vi "sinusiki 22.vi"(6 "k":dbl, 9 "N":i32, 10 "Faza":dbl, 11 "Amplituda":dbl) -> (3 "Array":dbl[](array[numeric]))   [LabVIEW 2020]
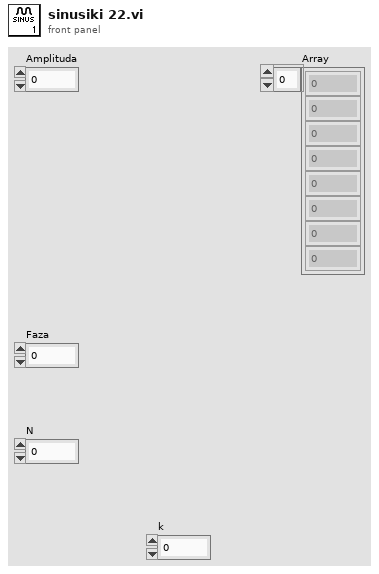
[diagram p1: front panel]
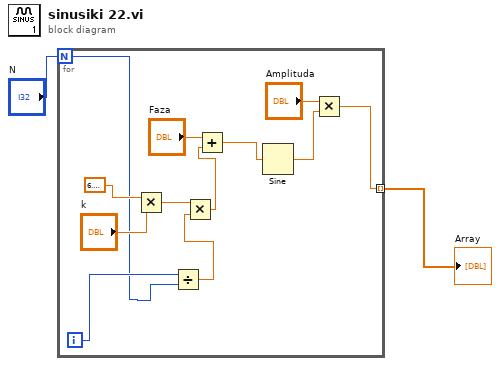
[diagram p0: block diagram]
diagram:
  n1 = for {
    N: "N" -> [w3]
    tunnel: [w11] -> w2 mode=indexing
    i -> [w14]
    n2 = Multiply(x=6.283185307179586, y="k") -> (x*y=w6:dbl)
    n3 = Divide(x=w14, y=w3) -> (x/y=w10:dbl)
    n4 = Multiply(x=w6, y=w10) -> (x*y=w9:dbl)
    n5 = Add(x="Faza", y=w9) -> (x+y=w8:dbl)
    n6 = Sine(x=w8) -> (sin(x)=w12:dbl)
    n7 = Multiply(x="Amplituda", y=w12) -> (x*y=w11:dbl)
  }
  "Array" <- w2
